vi "Teleop.vi"(10 "Match Info":T1={"Autonomous Elapsed Seconds"=0.0, "TeleOp Elapsed Seconds"=0.0, "Disabled Elapsed Seconds"=0.0, "Visited Autonomous"=FALSE, "Visited TeleOp"=FALSE, "Visited Disabled"=FALSE, "Autonomous Settings"={"Autonomous Style"=enum."Independent", "VI Refnum"=refnum}}, 11 "Call Context":T2) -> ()   [LabVIEW 2012]
doc: "This VI is called for each TeleOp packet received from the DS where the robot is not disabled. It is often used to read from the joysticks and update I/O or to update setpoints for timed control loops. It should complete and return within 20 milliseconds or it may miss DS packets."
uses:
  <vilib>/Rock Robotics/WPI/DriverStation/WPI_DriverStationDerivedRobotMode.ctl
  <vilib>/Rock Robotics/WPI/DriverStation/WPI_DriverStationMatch Info.ctl
  <vilib>/Rock Robotics/WPI/Solenoid/WPI_SolenoidValue.ctl
  Robot Global Data.vi
  <vilib>/Rock Robotics/WPI/Solenoid/WPI_SolenoidSetEnum.vi
panel:
  out "Loop Time 2":u32(graph)
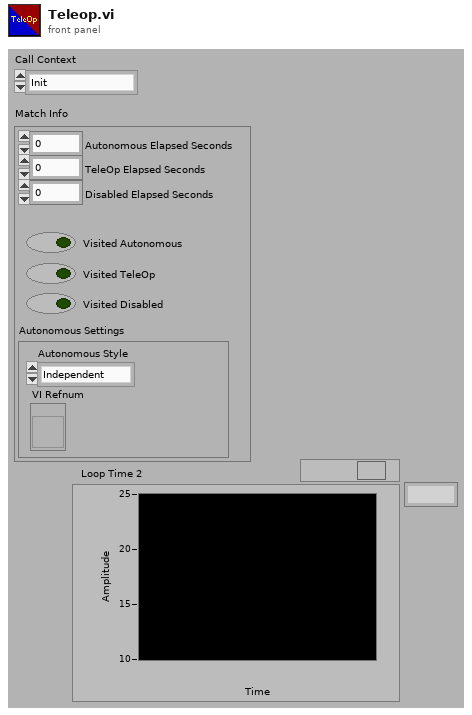
[diagram p1: front panel]
types:
  T1 = typedef "WPI_DriverStationMatch Info.ctl" = cluster{"Autonomous Elapsed Seconds":dbl, "TeleOp Elapsed Seconds":dbl, "Disabled Elapsed Seconds":dbl, "Visited Autonomous":bool, "Visited TeleOp":bool, "Visited Disabled":bool, "Autonomous Settings":cluster{"Autonomous Style":enum16{"Iterative", "Independent"}, "VI Refnum":refnum<vi>}}
  T2 = typedef "WPI_DriverStationDerivedRobotMode.ctl" = enum16{"Init", "Execute", "Stop"}
  T3 = typedef "WPI_SolenoidValue.ctl" = enum16{"Off", "On", "Forward", "Reverse"}
  T4 = cluster{"Shift Desired?":bool, "Precision Mode?":bool, "Forward-Back":dbl}
  T5 = cluster{"Precision Mode?":bool, "Left-Right":dbl, "Shift Desired":bool, "Manual Shooter Speed":dbl}
  T6 = cluster{"Run Shooter":bool, "Should Fire":bool, "Deploy Lifter":bool, "Spatula Toggle":bool, "Release Lifter":bool, "Override Shooter":bool, "Reset Lifter":bool, "Grab Left Frisbee":bool, "Grab Right Frisbee":bool, "n00b Toggle":bool}
  T7 = typedef "WPI_SolenoidDevRef.ctl" = cluster{"DevStatus":errorcluster, "Solenoid Module":T8, "Forward Solenoid Channel":T9, "Reverse Solenoid Channel":T9}
  T8 = typedef "FPGA_TypedefSolenoidModule.ctl" = enum16{"Solenoid Module 1", "Solenoid Module 2"}
  T9 = typedef "WPI_SolenoidChannel.ctl" = enum8{"Solenoid 1", "Solenoid 2", "Solenoid 3", "Solenoid 4", "Solenoid 5", "Solenoid 6", "Solenoid 7", "Solenoid 8", "Invalid"}
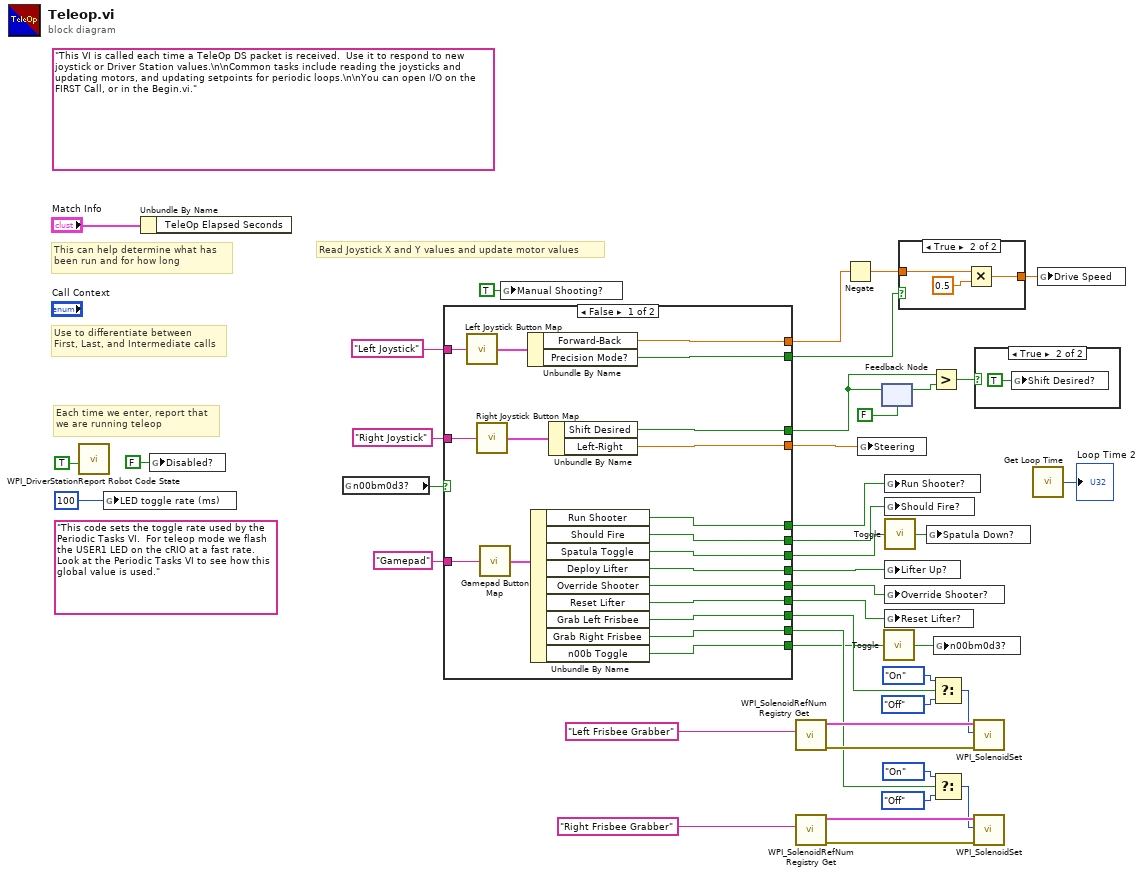
[diagram p0: block diagram]
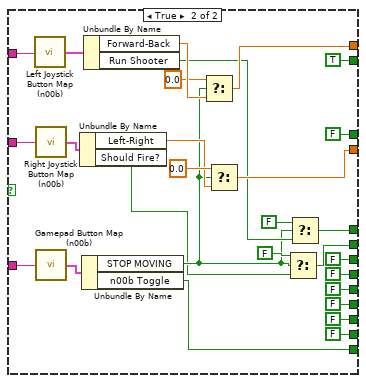
[diagram p2: hidden frame]
diagram:
  (unwired) "This code sets the toggle rate used by the Periodic Tasks VI.  For teleop mode we flash the USER1 LED on the cRIO at a fast rate.  Look at the Periodic Tasks VI to see how this global value is used."
  (unwired) "This VI is called each time a TeleOp DS packet is received.  Use it to respond to new joystick or Driver Station values.\n\nCommon tasks include reading the joysticks and updating motors, and updating setpoints for periodic loops.\n\nYou can open I/O on the FIRST Call, or in the Begin.vi."
  # "Each time we enter, report that\nwe are running teleop"
  # "Use to differentiate between\nFirst, Last, and Intermediate calls"
  # "This can help determine what has\nbeen run and for how long"
  # "Read Joystick X and Y values and update motor values"
  n1 = call <vilib>:"WPI_DriverStationReport Robot Code State.vi"("TeleOp"=TRUE ("Autonomous")) -> ()  [unwired: 10 in, 1 out]
  n2 = global write "Robot Global Data.vi" "LED toggle rate (ms)"(u32 100 ("LED ms toggle rate")) -> ()
  n3 = Unbundle By Name("Match Info") -> ()  [unwired: 1 out]
  n4 = global write "Robot Global Data.vi" "Disabled?"(FALSE ("Disabled?")) -> ()
  n5 = global read "Robot Global Data.vi" "n00bm0d3?"() -> (w6:bool)
  n6 = case shown="False" w6 {
    tunnel: [w59 w79] -> w35
    tunnel: [w58 w76] -> w33
    tunnel: [w56 w74] -> w32
    tunnel: [w55 w65] -> w31
    tunnel: [w54 FALSE ("Spatula Toggle")] -> w30
    tunnel: [w53 FALSE ("Override Shooter")] -> w28
    tunnel: [w52 TRUE ("Precision Mode?")] -> w27
    tunnel: [w51 FALSE ("Shift Desired")] -> w26
    tunnel: [w50 FALSE ("Deploy Lifter")] -> w23
    tunnel: [w49 FALSE ("Reset Lifter")] -> w22
    tunnel: [w48 FALSE ("Grab Left Frisbee")] -> w13
    tunnel: [w47 FALSE ("Grab Right Frisbee")] -> w7
    tunnel: "Gamepad" ("refnum name") -> [w46 w89]
    tunnel: "Right Joystick" ("refnum name") -> [w45 w88]
    tunnel: "Left Joystick" ("refnum name") -> [w44 w87]
    tunnel: [w43 w62] -> w1
    frame False {
      n7 = call "Left Joystick Button Map.vi"("Joystick Name"=w44) -> ("Actions"=w60:T4)
      n8 = call "Right Joystick Button Map.vi"("Joystick Name"=w45) -> ("Actions"=w61:T5)
      n9 = call "Gamepad Button Map.vi"("Joystick Name"=w46) -> ("Actions"=w57:T6)
      n10 = Unbundle By Name(w60) -> ("Forward-Back"=w59:dbl, "Precision Mode?"=w52:bool)
      n11 = Unbundle By Name(w57) -> ("Run Shooter"=w56:bool, "Should Fire"=w55:bool, "Spatula Toggle"=w54:bool, "Deploy Lifter"=w50:bool, "Override Shooter"=w53:bool, "Reset Lifter"=w49:bool, "Grab Left Frisbee"=w48:bool, "Grab Right Frisbee"=w47:bool, "n00b Toggle"=w43:bool)
      n12 = Unbundle By Name(w61) -> ("Shift Desired"=w51:bool, "Left-Right"=w58:dbl)
    }
    frame True {
      n13 = call "Left Joystick Button Map (n00b).vi"("Joystick Name"=w87) -> ("Actions"=w75:cluster{"Forward-Back":dbl, "Run Shooter":bool})
      n14 = call "Right Joystick Button Map (n00b).vi"("Joystick Name"=w88) -> ("Actions"=w84:cluster{"Left-Right":dbl, "Should Fire?":bool})
      n15 = call "Gamepad Button Map (n00b).vi"("Joystick Name"=w89) -> ("Actions"=w86:cluster{"STOP MOVING":bool, "n00b Toggle":bool})
      n16 = Unbundle By Name(w84) -> ("Left-Right"=w77:dbl, "Should Fire?"=w63:bool)
      n17 = Unbundle By Name(w86) -> ("STOP MOVING"=w64:bool, "n00b Toggle"=w62:bool)
      n18 = Unbundle By Name(w75) -> ("Forward-Back"=w81:dbl, "Run Shooter"=w72:bool)
      n19 = Select(t=0.0, s=w64, f=w81) -> (s? t:f=w79:dbl)
      n20 = Select(t=0.0, s=w64, f=w77) -> (s? t:f=w76:dbl)
      n21 = Select(t=FALSE ("Spatula Toggle"), s=w64, f=w63) -> (s? t:f=w65:bool)
      n22 = Select(t=FALSE ("Spatula Toggle"), s=w64, f=w72) -> (s? t:f=w74:bool)
    }
  }
  n23 = global write "Robot Global Data.vi" "Manual Shooting?"(TRUE ("Disabled?")) -> ()
  n24 = call <vilib>:"WPI_SolenoidRefNum Registry Get.vi"("refnum name"="Left Frisbee Grabber") -> ("error out"=w17:errorcluster, "SolenoidDevRef"=w18:T7)  [unwired: 9 in]
  n25 = call <vilib>:"WPI_SolenoidRefNum Registry Get.vi"("refnum name"="Right Frisbee Grabber") -> ("error out"=w15:errorcluster, "SolenoidDevRef"=w16:T7)  [unwired: 9 in]
  n26 = Negate(x=w35) -> (-x=w29:dbl)
  n27 = global write "Robot Global Data.vi" "Steering"(w33) -> ()
  n28 = feedback-in #1(w26) -> ()
  n29 = feedback #1(FALSE ("Shift Desired?")) -> (w38:bool)
  n30 = call "Toggle.vi"("Input"=w1) -> ("Output"=w2:bool)
  n31 = global write "Robot Global Data.vi" "Run Shooter?"(w32) -> ()
  n32 = global write "Robot Global Data.vi" "Should Fire?"(w31) -> ()
  n33 = call "Toggle.vi"("Input"=w30) -> ("Output"=w24:bool)
  n34 = global write "Robot Global Data.vi" "Lifter Up?"(w23) -> ()
  n35 = global write "Robot Global Data.vi" "Override Shooter?"(w28) -> ()
  n36 = global write "Robot Global Data.vi" "Reset Lifter?"(w22) -> ()
  n37 = case shown="True" w27 {
    tunnel: w29 -> [w90 w93]
    tunnel: [w90 w91] -> w34
    frame False {
    }
    frame True {
      n38 = Multiply(x=w93, y=0.5) -> (x*y=w91:dbl)
    }
  }
  n39 = global write "Robot Global Data.vi" "Spatula Down?"(w24) -> ()
  n40 = Greater?(x=w26, y=w38) -> (0:w37:bool)
  n41 = Select(t=WPI_SolenoidValue."On" ("Value"), s=w13, f=WPI_SolenoidValue."Off" ("Value")) -> (s? t:f=w11:T3)
  n42 = Select(t=WPI_SolenoidValue."On" ("Value"), s=w7, f=WPI_SolenoidValue."Off" ("Value")) -> (s? t:f=w8:T3)
  n43 = global write "Robot Global Data.vi" "n00bm0d3?"(w2) -> ()
  n44 = call-poly <vilib>:"WPI_SolenoidSet.vi"("error in (no error)"=w17, "Value"=w11, "SolenoidDevRef"=w18) -> ()  [unwired: 7 in, 2 out]
  n45 = call-poly <vilib>:"WPI_SolenoidSet.vi"("error in (no error)"=w15, "Value"=w8, "SolenoidDevRef"=w16) -> ()  [unwired: 7 in, 2 out]
  n46 = case shown="True" w37 {
    frame False {
    }
    frame True {
      n47 = global write "Robot Global Data.vi" "Shift Desired?"(TRUE ("Shift Desired?")) -> ()
    }
  }
  n48 = call "Get Loop Time.vi"() -> ("Loop Time"=→"Loop Time 2":u32)  [unwired: 1 in]
  n49 = global write "Robot Global Data.vi" "Drive Speed"(w34) -> ()
